vi "new  process file.vi"() -> ()   [LabVIEW 2018]
panel:
  in  "process name":string
  out "count":dbl
  out "multiple":string
  out "single":string
  in  "SEARCH":bool
  in  "EXIT":bool
  in  "SAVE":bool
  in  "DELETE":bool
  in  "ADD":bool
  # "Process Name"
  # "Recipe Name"
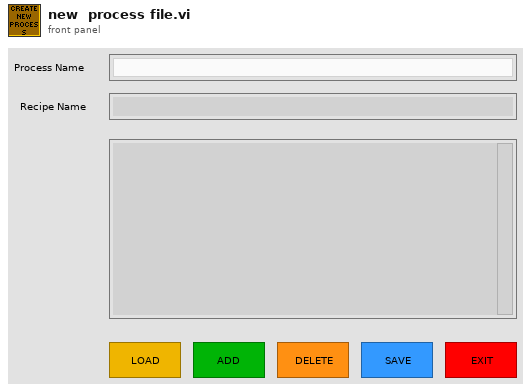
[diagram p1: front panel]
types:
  T1 = enum16{"open", "replace", "create", "open or create", "replace or create", "replace or create with confirmation"}
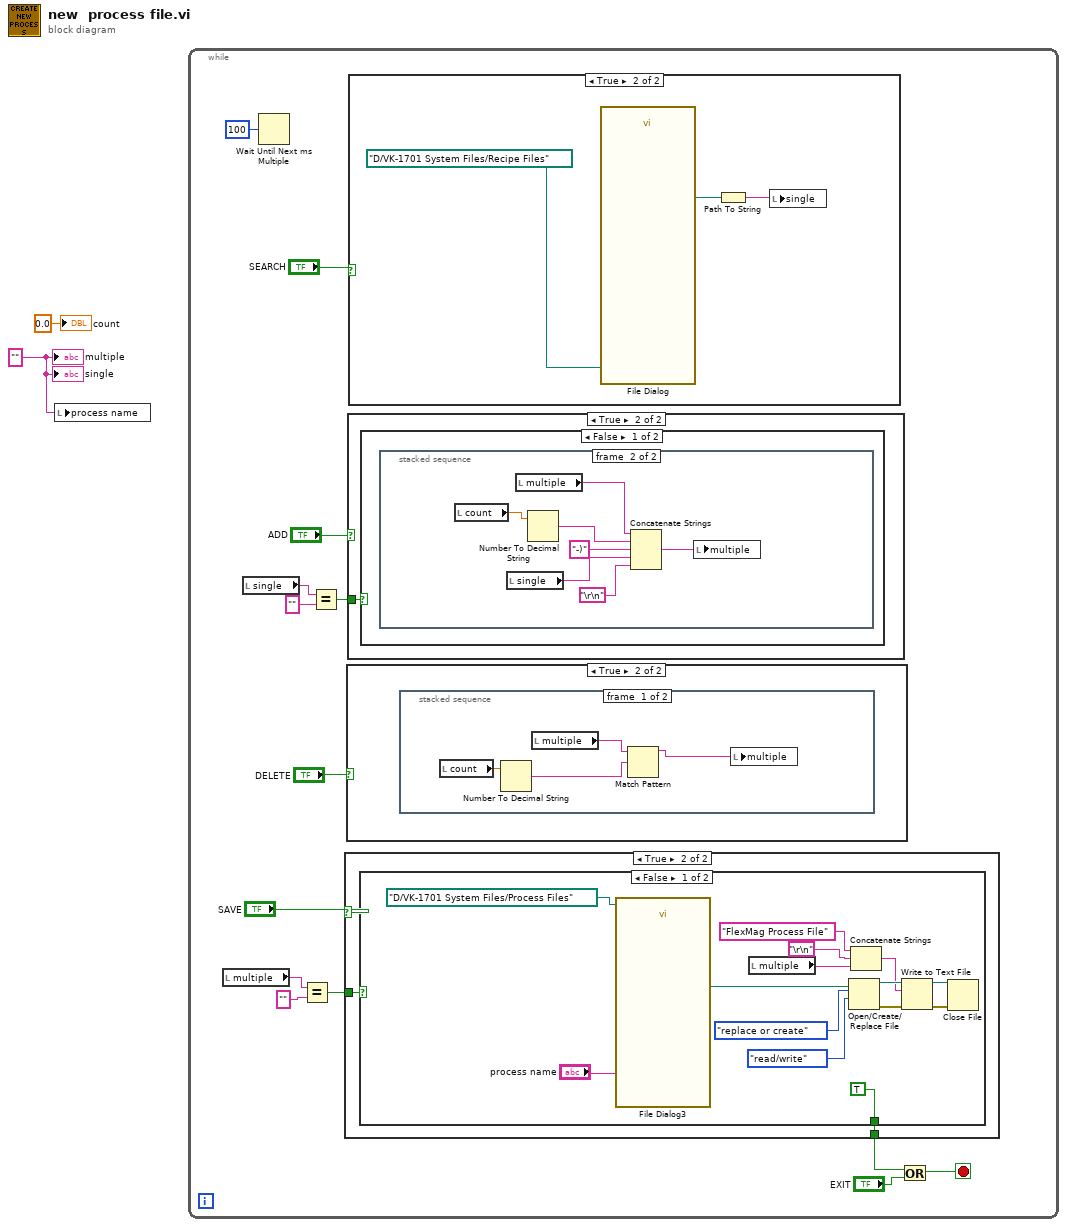
[diagram p0: block diagram]
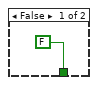
[diagram p2: hidden frame]
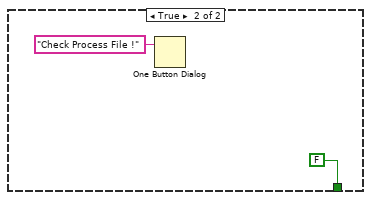
[diagram p3: hidden frame]
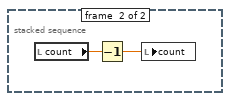
[diagram p5: hidden frame]
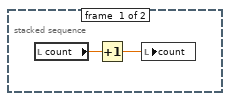
[diagram p7: hidden frame]
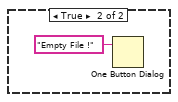
[diagram p8: hidden frame]
diagram:
  w1 = "" ("multiple")
  n1 = local write "process name"(w1) -> ()
  n2 = while {
    stop <- w3 stop-if-true
    n3 = local read "multiple"() -> (w7:string)
    n4 = local read "single"() -> (w14:string)
    n5 = Wait Until Next ms Multiple(millisecond multiple=u32 100) -> ()  [unwired: 1 out]
    n6 = Equal?(x=w7, y="") -> (x = y?=w6:bool)
    n7 = Equal?(x=w14, y="") -> (x = y?=w12:bool)
    n8 = case shown="True" "SAVE" {
      tunnel: w6 -> [_ w19]
      tunnel: [FALSE w18] -> w4
      frame False {
      }
      frame True {
        n9 = case shown="False" w19 {
          tunnel: [TRUE FALSE] -> w18
          frame False {
            n10 = call "File Dialog3"("start path"=path "D:/VK-1701 System Files/Process Files", "default name"="process name") -> ("selected path"=w29:path)  [unwired: 10 in, 3 out]
            n11 = local read "multiple"() -> (w22:string)
            n12 = Open/Create/Replace File(file path (use dialog)=w29, operation (0:open)=T1."replace or create", access (0:read/write)=enum16{"read/write", "read-only", "write-only"}."read/write") -> (refnum out=w26:refnum<file>, error out=w25:errorcluster)  [unwired: 3 in, 1 out]
            n13 = Concatenate Strings("FlexMag Process File" ("y"), "\r\n", w22) -> (w23:string)
            n14 = Write to Text File(file (use dialog)=w26, text=w23, error in=w25) -> (refnum out=w28:refnum<file>, error out=w27:errorcluster)  [unwired: 1 in, 1 out]
            n15 = Close File(refnum=w28, error in=w27) -> ()  [unwired: 2 out]
          }
          frame True {
            n16 = One Button Dialog(message="Check Process File !") -> ()  [unwired: 1 in, 1 out]
          }
        }
      }
    }
    n17 = case shown="True" "DELETE" {
      frame False {
      }
      frame True {
        n18 = stacked-sequence {
          frame #0 {
            n19 = local read "count"() -> (w39:dbl)
            n20 = Number To Decimal String(number=w39) -> (decimal integer string=w37:string)  [unwired: 1 in]
            n21 = local read "multiple"() -> (w38:string)
            n22 = Match Pattern(string=w38, regular expression=w37) -> (before substring=w36:string)  [unwired: 1 in, 3 out]
            n23 = local write "multiple"(w36) -> ()
          }
          frame #1 {
            n24 = local read "count"() -> (w41:dbl)
            n25 = Decrement(x=w41) -> (x-1=w40:dbl)
            n26 = local write "count"(w40) -> ()
          }
        }
      }
    }
    n27 = case shown="True" "ADD" {
      tunnel: w12 -> [_ w42]
      frame False {
      }
      frame True {
        n28 = case shown="False" w42 {
          frame False {
            n29 = stacked-sequence {
              frame #0 {
                n30 = local read "count"() -> (w43:dbl)
                n31 = Increment(x=w43) -> (x+1=w44:dbl)
                n32 = local write "count"(w44) -> ()
              }
              frame #1 {
                n33 = local read "count"() -> (w51:dbl)
                n34 = local read "single"() -> (w48:string)
                n35 = local read "multiple"() -> (w46:string)
                n36 = Number To Decimal String(number=w51) -> (decimal integer string=w50:string)  [unwired: 1 in]
                n37 = Concatenate Strings(w46, w50, "-)" ("string"), w48, "\r\n") -> (w47:string)
                n38 = local write "multiple"(w47) -> ()
              }
            }
          }
          frame True {
            n39 = One Button Dialog(message="Empty File !") -> ()  [unwired: 1 in, 1 out]
          }
        }
      }
    }
    n40 = case shown="True" "SEARCH" {
      frame False {
      }
      frame True {
        n41 = call "File Dialog"("start path"=path "D:/VK-1701 System Files/Recipe Files") -> ("selected path"=w54:path)  [unwired: 11 in, 3 out]
        n42 = Path To String(path=w54) -> (string=w53:string)
        n43 = local write "single"(w53) -> ()
      }
    }
    n44 = Or(x=w4, y="EXIT") -> (x .or. y?=w3:bool)
  }
  "multiple" <- w1
  "count" <- 0.0 ("count")
  "single" <- w1
